vi "Autonomous.vi"() -> ()   [LabVIEW 2020]
doc: "This VI starts when autonomous period begins, and will automatically be terminated when it ends. You can carry out timed or sensor driven operations directly to I/O or to subsystems without needing to return to the caller."
uses:
  manipulator/Implementation/Typedefs/game object.ctl
  <vilib>/Rock Robotics/WPI/Utilities/WPI_GetSetVariantRefNum.vi
  <vilib>/Rock Robotics/Network Tables/NT Read Boolean.vi
  Framework/Robot Global Data.vi
  <vilib>/Rock Robotics/Network Tables/NT Read String Array.vi
  <vilib>/Rock Robotics/Network Tables/NT Read Number.vi
panel:
  in  "Is Blue Alliance?":bool=TRUE
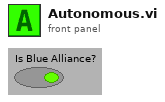
[diagram p1: front panel]
types:
  T1 = typedef "WPI_JoystickDevRef.ctl" = cluster{"Device":T2}
  T2 = typedef "WPI_JoystickDeviceEnum.ctl" = enum16{"USB 0", "USB 1", "USB 2", "USB 3", "USB 4", "USB 5"}
  T3 = typedef "game object.ctl" = enum16{"Nothing", "Cone", "Cube"}
  T4 = cluster{"Field Centric?":bool, "SnapToScore":bool, "TranslationalAlign":bool}
  T5 = typedef "Robot Velocities.ctl" = cluster{"X Velocity":dbl, "Y Velocity":dbl, "Rotational \nVelocity":dbl}
  T6 = typedef "Single Cmd Info.ctl" = cluster{"Name":string, "CPTM.DataType":variant, "All Control Values Variant":cluster{"Name":string, "Variant Data":variant}[], "icon full":T7, "icon scaled":T7, "Path":path, "Subsystem Color":u32}
  T7 = typedef "imagedata.ctl" = cluster{"image type":i32, "image depth":i32, "image":u8[], "mask":u8[], "colors":u32[], "Rectangle":cluster{"left":i16, "top":i16, "right":i16, "bottom":i16}}
  T8 = cluster{"Name":string, "vi reference":refnum<vi>, i32[], variant[]}
  T9 = cluster{dbl, "Command out":cluster{"Name":string, "vi reference":refnum<vi>, i32[], variant[]}}
  T10 = cluster{dbl, "Command out":cluster{"Name":string, "vi reference":refnum<vi>, i32[], variant[]}}[]
  T11 = cluster{"Velocities":T5[], "Positions":cluster{"x":dbl, "y":dbl, "th":dbl}[], cluster{dbl, "Command out":cluster{"Name":string, "vi reference":refnum<vi>, i32[], variant[]}}[], "Zero Velocity?":bool[]}
  T12 = typedef "CTRE_PigeonIMU_DeviceRef.ctl" = cluster{"DeviceStatus":errorcluster, "Device Number":u8, "Type":T13, "Device ID":u32, "Handle":u64, "UsageFrame":u32, "Library Path":path}
  T13 = typedef "CTRE_PigeonIMU_ConnectionType.ctl" = u32
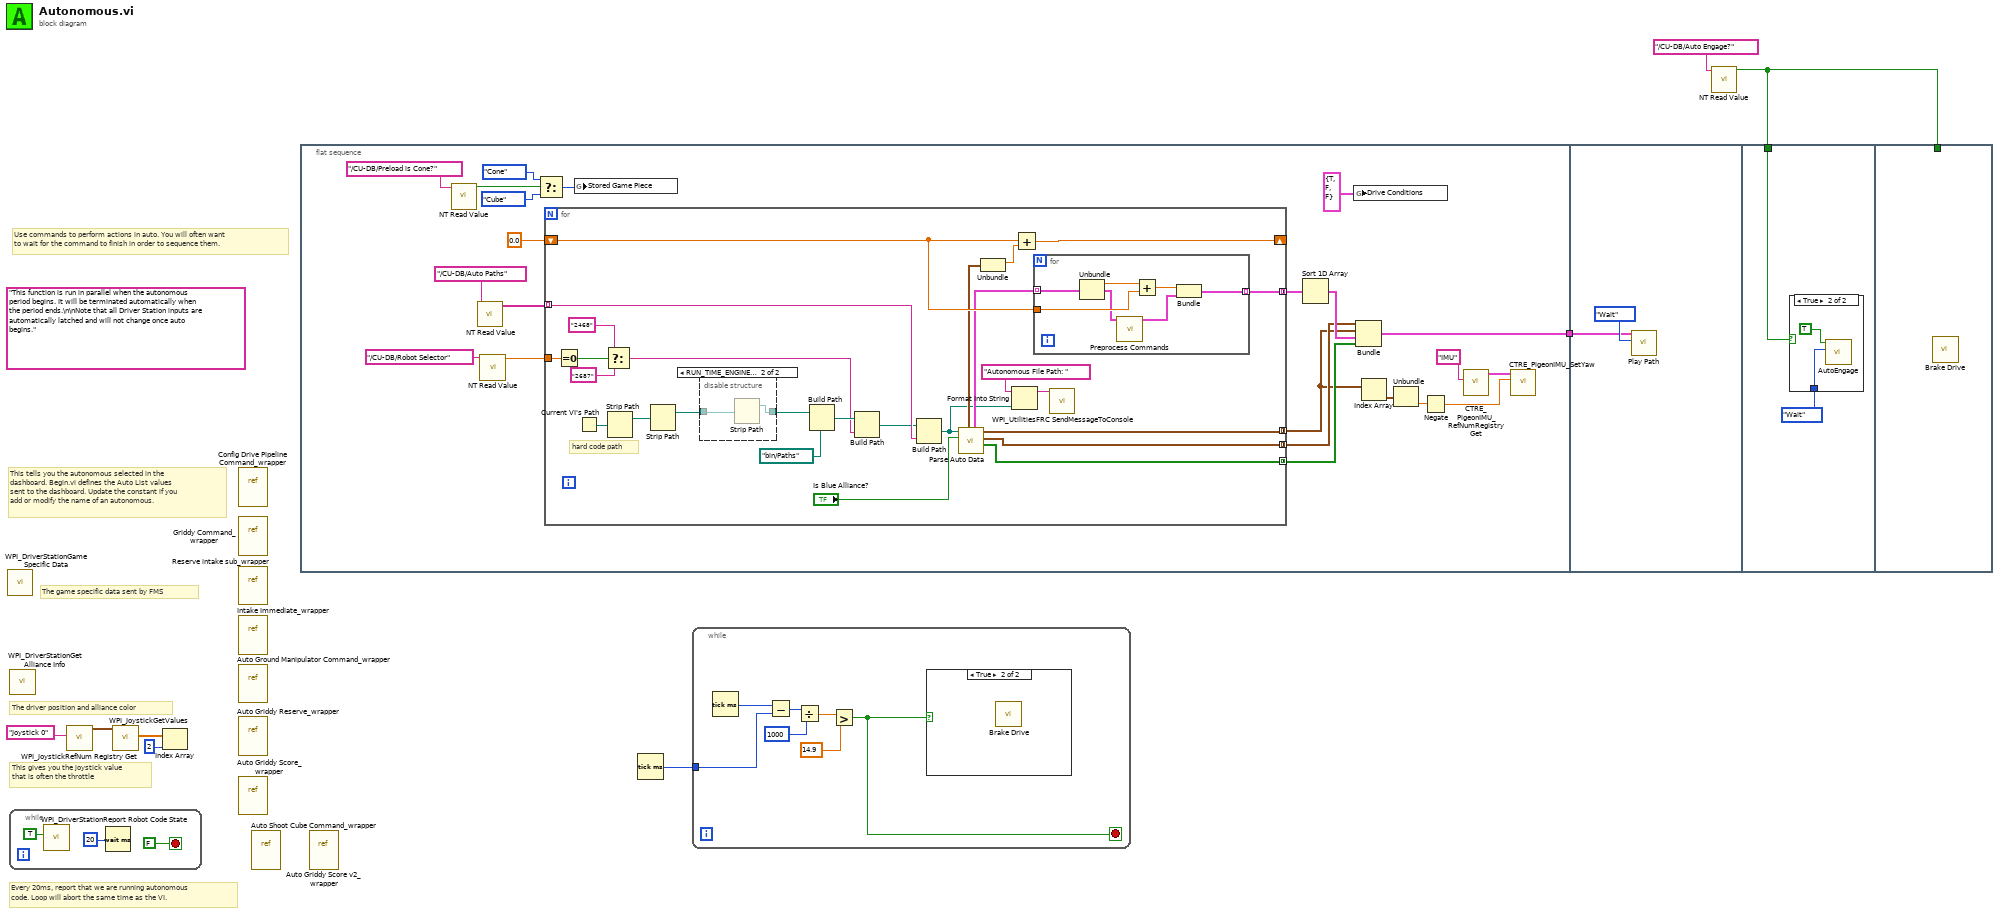
[diagram p0: block diagram]
diagram:
  (unwired) "This function is run in parallel when the autonomous period begins. It will be terminated automatically when the period ends.\n\nNote that all Driver Station inputs are automatically latched and will not change once auto begins."
  # "The game specific data sent by FMS"
  # "This tells you the autonomous selected in the \ndashboard. Begin.vi defines the Auto List values\nsent to the dashboard. Update the constant if you\nadd or modify the name of an autonomous."
  # "Every 20ms, report that we are running autonomous\ncode. Loop will abort the same time as the VI."
  # "This gives you the joystick value\nthat is often the throttle"
  # "Use commands to perform actions in auto. You will often want\nto wait for the command to finish in order to sequence them."
  # "The driver position and alliance color"
  n1 = call <vilib>:"WPI_DriverStationGame Specific Data.vi"() -> ()  [unwired: 11 in, 1 out]
  n2 = while {
    stop <- FALSE stop-if-true
    n3 = call <vilib>:"WPI_DriverStationReport Robot Code State.vi"("Autonomous"=TRUE) -> ()  [unwired: 10 in, 1 out]
    n4 = Wait (ms)(milliseconds to wait=u32 20) -> ()  [unwired: 1 out]
  }
  n5 = call <vilib>:"WPI_DriverStationGet Alliance Info.vi"() -> ()  [unwired: 12 out]
  n6 = call <vilib>:"WPI_JoystickRefNum Registry Get.vi"("refnum name"="Joystick 0") -> ("JoystickDevRef"=w7:T1)  [unwired: 1 in, 9 out]
  n7 = call <vilib>:"WPI_JoystickGetValues.vi"("JoystickDevRef"=w7) -> ("Axes"=w6:dbl[])  [unwired: 6 in, 4 out]
  n8 = Index Array(array=w6, index=2) -> ()  [unwired: 1 out]
  n9 = vi-ref "Config Drive Pipeline Command_wrapper.vi"() -> ()  [unwired: 1 out]
  n10 = vi-ref "Griddy Command_wrapper.vi"() -> ()  [unwired: 1 out]
  n11 = vi-ref "Reserve intake sub_wrapper.vi"() -> ()  [unwired: 1 out]
  n12 = vi-ref "Intake Immediate_wrapper.vi"() -> ()  [unwired: 1 out]
  n13 = vi-ref "Auto Ground Manipulator Command_wrapper.vi"() -> ()  [unwired: 1 out]
  n14 = vi-ref "Auto Griddy Reserve_wrapper.vi"() -> ()  [unwired: 1 out]
  n15 = vi-ref "Auto Griddy Score_wrapper.vi"() -> ()  [unwired: 1 out]
  n16 = vi-ref "Auto Shoot Cube Command_wrapper.vi"() -> ()  [unwired: 1 out]
  n17 = flat-sequence {
    tunnel: [w21] -> w4
    tunnel: w4 -> [w70]
    tunnel: w2 -> [w73]
    tunnel: w2 -> [_]
    frame #0 {
      n18 = call-poly <vilib>:"NT Read Value.vi"("name"="/CU-DB/Preload is Cone?") -> ("value"=w15:bool)  [unwired: 8 in, 2 out]
      n19 = call-poly <vilib>:"NT Read Value.vi"("name"="/CU-DB/Auto Paths") -> ("value"=w28:string[])  [unwired: 8 in, 2 out]
      n20 = call-poly <vilib>:"NT Read Value.vi"("name"="/CU-DB/Robot Selector") -> ("value"=w19:dbl)  [unwired: 8 in, 2 out]
      n21 = Select(t=game_object."Cone" ("Stored Game Piece"), s=w15, f=game_object."Cube" ("Stored Game Piece")) -> (s? t:f=w12:T3)
      n22 = for {
        tunnel: [w47] -> w18 mode=concatenating
        tunnel: [w48] -> w17 mode=concatenating
        shift-right: [w53] -> _
        shift-left: 0.0 -> [w51]
        tunnel: [w52] -> w30 mode=concatenating
        tunnel: [w37] -> w22 mode=concatenating
        tunnel: w28 -> [w46] mode=indexing
        tunnel: w19 -> [w43]
        # "hard code path"
        n23 = Equal To 0?(x=w43) -> (x = 0?=w42:bool)
        n24 = Current VI's Path() -> (path=w56:path)
        n25 = Select(t="2468", s=w42, f="2687") -> (s? t:f=w39:string)
        n26 = Strip Path(path=w56) -> (stripped path=w57:path)  [unwired: 1 out]
        n27 = Strip Path(path=w57) -> (stripped path=w59:path)  [unwired: 1 out]
        n28 = disable-structure shown="RUN_TIME_ENGINE==True, Default" {
          disable-tunnel: [w67 w68] -> w58
          disable-tunnel: w59 -> [w67 w69]
          frame condition #0 (active) {
          }
          frame condition #1 {
            n29 = Strip Path(path=w69) -> (stripped path=w68:path)  [unwired: 1 out]
          }
        }
        n30 = Build Path(base path=w58, name or relative path=path "bin/Paths") -> (appended path=w45:path)
        n31 = Build Path(base path=w45, name or relative path=w39) -> (appended path=w44:path)
        n32 = Build Path(base path=w44, name or relative path=w46) -> (appended path=w36:path)
        n33 = call "Parse Auto Data.vi"("Is Blue Alliance?"="Is Blue Alliance?", "path"=w36) -> ("Zero Velocity?"=w37:bool[], "Velocities"=w47:T5[], "Positions"=w48:cluster{"x":dbl, "y":dbl, "th":dbl}[], "Commands out"=w38:cluster{"Time (s)":dbl, T6, bool}[], "Overall"=w50:cluster{"Time (s)":dbl, "Distance (ft)":dbl})  [unwired: 5 in]
        n34 = Unbundle(w50) -> ("Time (s)"=w54:dbl)  [unwired: 1 out]
        n35 = Format Into String(initial string="Autonomous File Path: ", w36) -> (resulting string=w35:string)  [unwired: 2 in, 1 out]
        n36 = Add(x=w51, y=w54) -> (x+y=w53:dbl)
        n37 = for {
          tunnel: w51 -> [w65]
          tunnel: w38 -> [w64] mode=indexing
          tunnel: [w60] -> w52 mode=indexing
          n38 = Unbundle(w64) -> ("Time (s)"=w66:dbl, w63:T6)  [unwired: 1 out]
          n39 = call "Preprocess Commands.vi"("Command In"=w63) -> ("Command out"=w61:T8)  [unwired: 10 in]
          n40 = Add(x=w66, y=w65) -> (x+y=w62:dbl)
          n41 = Bundle(w62, "Command out"=w61) -> (w60:T9)  [unwired: 1 in]
        }
        n42 = call <vilib>:"WPI_UtilitiesFRC SendMessageToConsole.vi"("Message"=w35) -> ()  [unwired: 14 in, 1 out]
      }
      n43 = global write "Robot Global Data.vi" "Stored Game Piece"(w12) -> ()
      n44 = Sort 1D Array(array=w30) -> (sorted array=w23:T10)
      n45 = global write "Robot Global Data.vi" "Drive Conditions"(T4 {"Field Centric?"=TRUE, "SnapToScore"=FALSE, "TranslationalAlign"=FALSE} ("Drive Conditions")) -> ()
      n46 = Bundle("Velocities"=w18, "Positions"=w17, w23, "Zero Velocity?"=w22) -> (w21:T11)  [unwired: 1 in]
      n47 = Index Array(array=w17) -> (element=w26:cluster{"x":dbl, "y":dbl, "th":dbl})  [unwired: 1 in]
      n48 = Unbundle(w26) -> ("th"=w25:dbl)  [unwired: 2 out]
      n49 = Negate(x=w25) -> (-x=w24:dbl)
      n50 = call <vilib>:"CTRE_PigeonIMU_RefNumRegistryGet.vi"("refnum name"="IMU") -> ("PigeonIMUDevRef"=w33:T12)  [unwired: 9 in, 1 out]
      n51 = call <vilib>:"CTRE_PigeonIMU_SetYaw.vi"("Value"=w24, "PigeonIMUDevRef"=w33) -> ()  [unwired: 8 in, 2 out]
    }
    frame #1 {
      n52 = call "Play Path.vi"("Synchronization"=enum16{"Start", "Wait"}."Wait", "Auto Data"=w70) -> ()  [unwired: 9 in, 1 out]
    }
    frame #2 {
      n53 = case shown="True" w73 {
        tunnel: enum16{"Start", "Wait"}."Wait" ("Synchronication") -> [_ w74]
        frame False {
        }
        frame True {
          n54 = call "AutoEngage.vi"("Synchronication"=w74, "Auto Engage Heading"=TRUE) -> ()  [unwired: 9 in, 1 out]
        }
      }
    }
    frame #3 {
      n55 = call "Brake Drive.vi"() -> ()  [unwired: 11 in, 1 out]
    }
  }
  n56 = vi-ref "Auto Griddy Score v2_wrapper.vi"() -> ()  [unwired: 1 out]
  n57 = Tick Count (ms)() -> (millisecond timer value=w1:u32)
  n58 = while {
    tunnel: w1 -> [w81]
    stop <- w76 stop-if-true
    n59 = Tick Count (ms)() -> (millisecond timer value=w82:u32)
    n60 = Subtract(x=w82, y=w81) -> (x-y=w80:u32)
    n61 = Divide(x=w80, y=u32 1000) -> (x/y=w78:dbl)
    n62 = Greater?(x=w78, y=14.9) -> (0:w76:bool)
    n63 = case shown="True" w76 {
      frame False {
      }
      frame True {
        n64 = call "Brake Drive.vi"() -> ()  [unwired: 11 in, 1 out]
      }
    }
  }
  n65 = call-poly <vilib>:"NT Read Value.vi"("name"="/CU-DB/Auto Engage?") -> ("value"=w2:bool)  [unwired: 8 in, 2 out]
